vi "Check Control Key.vi"(1 "Char":i16, 2 "VKey":T1) -> (0 "Control Key":T2)   [LabVIEW 2021, in "Seq Edit Quick Drop.lvlib"]
uses:
  Seq Edit Quick Drop.lvlib
  Control Keys.ctl
  <vilib>/event_ctls.llb/eventvkey.ctl
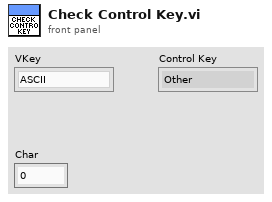
[diagram p1: front panel]
types:
  T1 = typedef "eventvkey.ctl" = enum16{"ASCII", "Enter", "Return", "Shift", "Ctrl", "Alt", "Cmd", "Opt", "Caps", "NumLock", "Clear", "Break", "Up", "Down", "Left", "Right", "Insert", "Delete", "Home", "End", "PageUp", "PageDown", "Escape", "Help", "Pause", "ScrollLock", "F1", "F2", "F3", "F4", "F5", "F6", "F7", "F8", "F9", "F10", "F11", "F12", "F13", "F14", "F15", "F16", "F17", "F18", "F19", "F20", "F21", "F22", "F23", "F24", "Play", "VolumeUp", "VolumeDown", "Mute", "Two Byte Char"}
  T2 = typedef "Seq Edit Quick Drop.lvlib/Control Keys.ctl" = enum16{"Other", "Enter", "Escape", "Tab", "Up", "Down"}
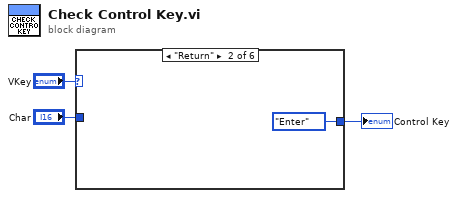
[diagram p0: block diagram]
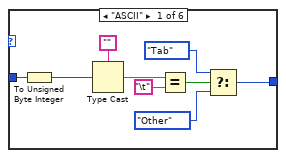
[diagram p2: hidden frame]
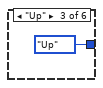
[diagram p3: hidden frame]
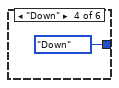
[diagram p4: hidden frame]
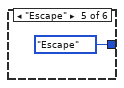
[diagram p5: hidden frame]
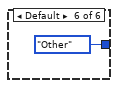
[diagram p6: hidden frame]
diagram:
  n1 = case shown="\"Return\"" "VKey" {
    tunnel: "Char" -> [w11 _ _ _ _ _]
    tunnel: [w4 Control_Keys."Enter" Control_Keys."Up" Control_Keys."Down" Control_Keys."Escape" Control_Keys."Other"] -> w3
    frame "ASCII" {
      n2 = To Unsigned Byte Integer(number=w11) -> (unsigned 8bit integer=w10:u8)
      n3 = Type Cast(type="", x=w10) -> (*(type *) &x=w9:string)
      n4 = Equal?(x=w9, y="\t") -> (x = y?=w7:bool)
      n5 = Select(t=Control_Keys."Tab", s=w7, f=Control_Keys."Other") -> (s? t:f=w4:T2)
    }
    frame "Return" {
    }
    frame "Up" {
    }
    frame "Down" {
    }
    frame "Escape" {
    }
    frame Default {
    }
  }
  "Control Key" <- w3
